vi "写入加标体积.vi"(7 "加标体积":dbl, 8 "error in (no error)":errorcluster caption="错误输入（无错误）", 11 "参数":enum16{"氨氮", "总磷", "总氮", "CODMn", "CODcr"}(ring)) -> (0 "error out":errorcluster caption="错误输出")   [LabVIEW 2016]
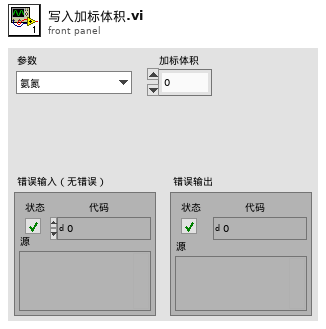
[diagram p1: front panel]
types:
  T1 = cluster{"氨氮":u8, "总磷":u8, "总氮":u8, "CODMn":u8, "CODCr":u8}
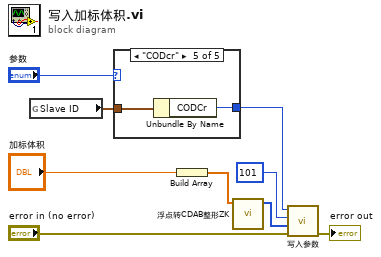
[diagram p0: block diagram]
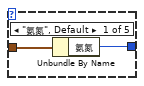
[diagram p2: hidden frame]
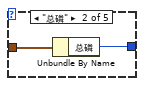
[diagram p3: hidden frame]
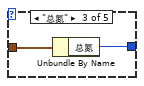
[diagram p4: hidden frame]
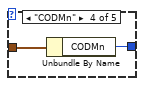
[diagram p5: hidden frame]
diagram:
  n1 = global read "断电保存全局.vi" "Slave ID"() -> (w5:T1)
  n2 = case shown="\"CODcr\"" "参数" {
    tunnel: w5 -> [w11 w13 w15 w17 w19]
    tunnel: [w10 w12 w14 w16 w18] -> w3
    frame "氨氮", Default {
      n3 = Unbundle By Name(w11) -> ("氨氮"=w10:u8)
    }
    frame "总磷" {
      n4 = Unbundle By Name(w13) -> ("总磷"=w12:u8)
    }
    frame "总氮" {
      n5 = Unbundle By Name(w15) -> ("总氮"=w14:u8)
    }
    frame "CODMn" {
      n6 = Unbundle By Name(w17) -> ("CODMn"=w16:u8)
    }
    frame "CODcr" {
      n7 = Unbundle By Name(w19) -> ("CODCr"=w18:u8)
    }
  }
  n8 = Build Array("加标体积") -> (w9:dbl[])
  n9 = call "浮点转CDAB整形ZK.vi"("浮点数"=w9) -> ("CDAB整形输出"=w7:u16[])  [unwired: 10 in]
  n10 = call "写入参数.vi"("Error in"="error in (no error)", "values"=w7, "starting address"=u16 101, "Slave ID"=w3) -> ("error out"=→"error out":errorcluster)  [unwired: 7 in]
